vi "fasad.vi"(0 "Data In":T4, 2 "Display State In":T2, 3 "Container State":T3) -> (6 "Data Out":T4, 7 "Display State Out":T2, 8 "Action":T1)   [LabVIEW 2019, in "Visual.xctl"]
uses:
  Visual.xctl
  data.ctl
  <vilib>/_xctls/Container State.ctl
  state.ctl
  <vilib>/_xctls/Action.ctl
  <vilib>/express/express analysis/Spectral/Block/exnSpectralBlock spectral measurements RMS poly.vi
  <vilib>/express/express analysis/Spectral/Block/exnSpectralBlock spectral measurements RMS WFM.vi
  <vilib>/express/express analysis/Spectral/XNode/ExpressSpectralMeasurementsBlockNode.xnode
  <vilib>/_xctls/XControlSupport.lvlib
panel:
  in  "Tab Control":enum32{"Page 1", "Page 2"}(tab)
  out "Digital Waveform Graph":digitalwaveform(graph)
  out "Analyzer":cluster{"f0":dbl, "df":dbl, "magnitude":dbl[]}(graph)
  out "Osciloscope":waveform(dbl)(graph)
  in  "Tree":string(tree)
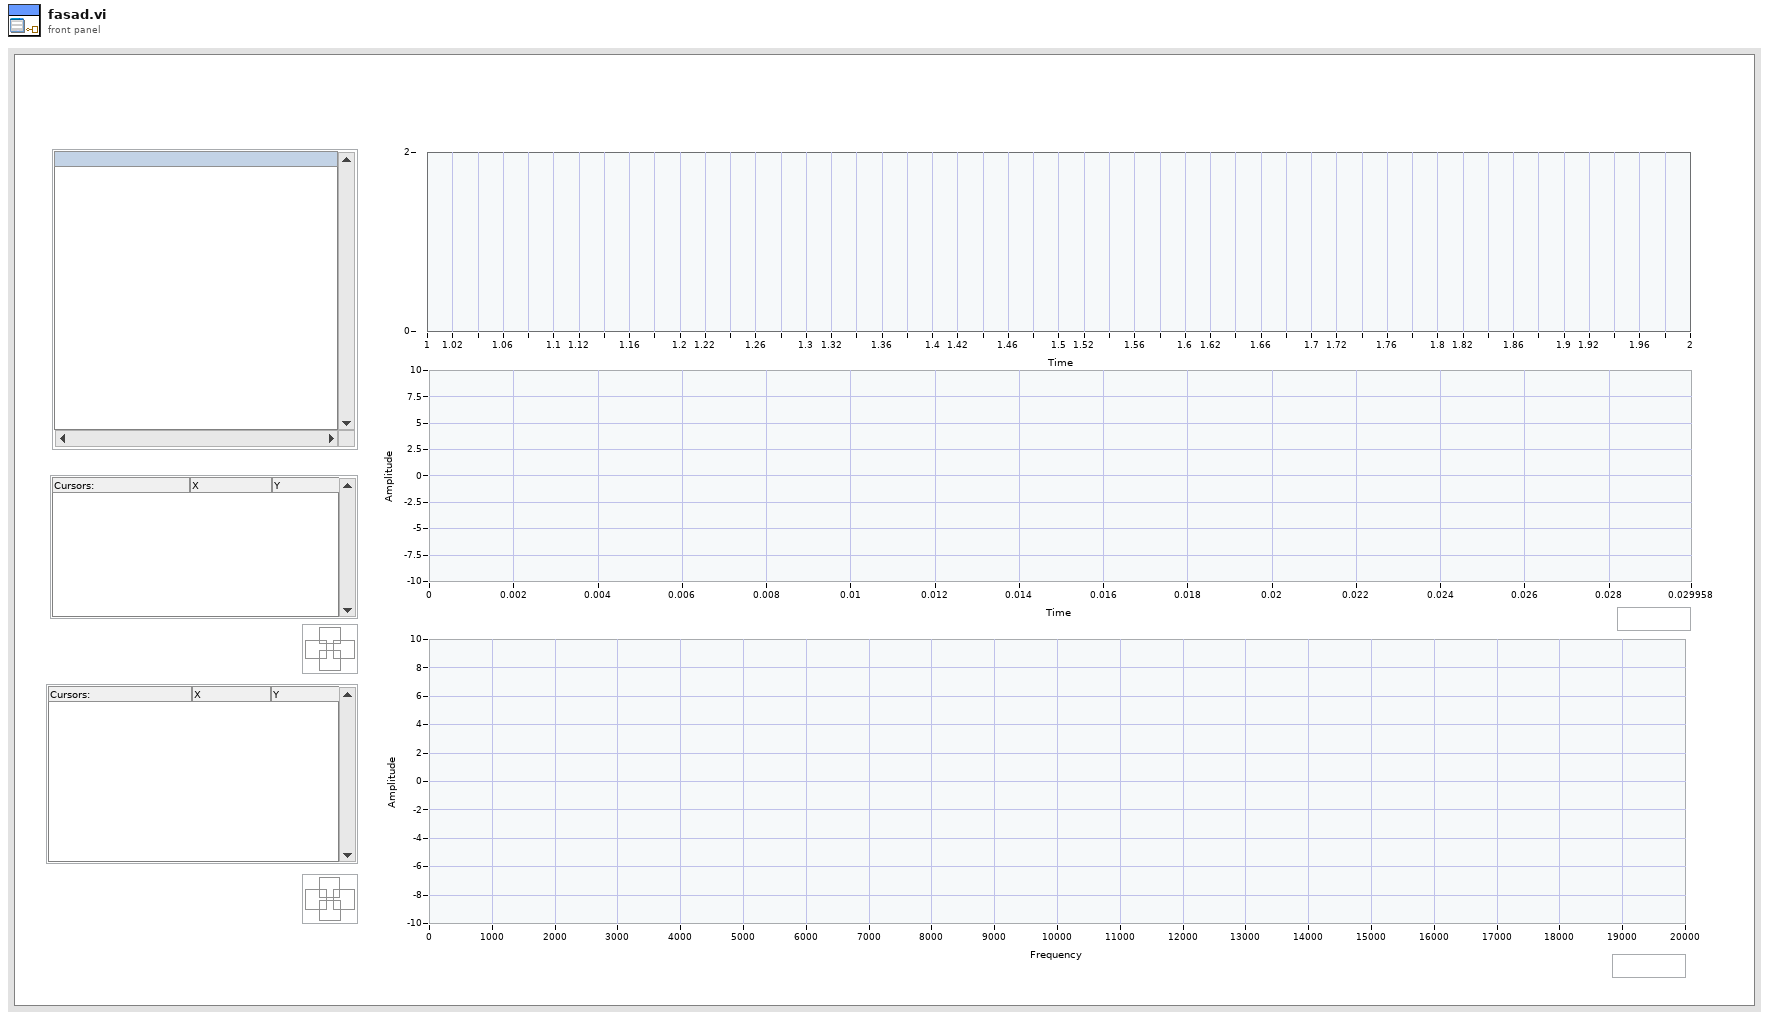
[diagram p1: front panel]
types:
  T1 = typedef "XControlSupport.lvlib/Action.ctl" = cluster{"Data Changed?":bool, "State Changed?":bool, "Action Name":string}
  T2 = typedef "Visual.xctl/state.ctl" = cluster{"Tree":string}
  T3 = typedef "XControlSupport.lvlib/Container State.ctl" = cluster{"Indicator?":bool, "Run Mode?":bool, " Refnum":refnum<vi>}
  T4 = typedef "Visual.xctl/data.ctl" = cluster{"Notes":string[], "Frame":u8[]}
  T5 = cluster{"averaging mode":u16, "weighting mode":u16, "number of averages":u32}
  T6 = cluster{"dB On (F)":bool, "unwrap phase (F)":bool, "convert to degree (F)":bool}
  T7 = enum8{"Enabled", "Disabled", "Disabled and Grayed Out"}
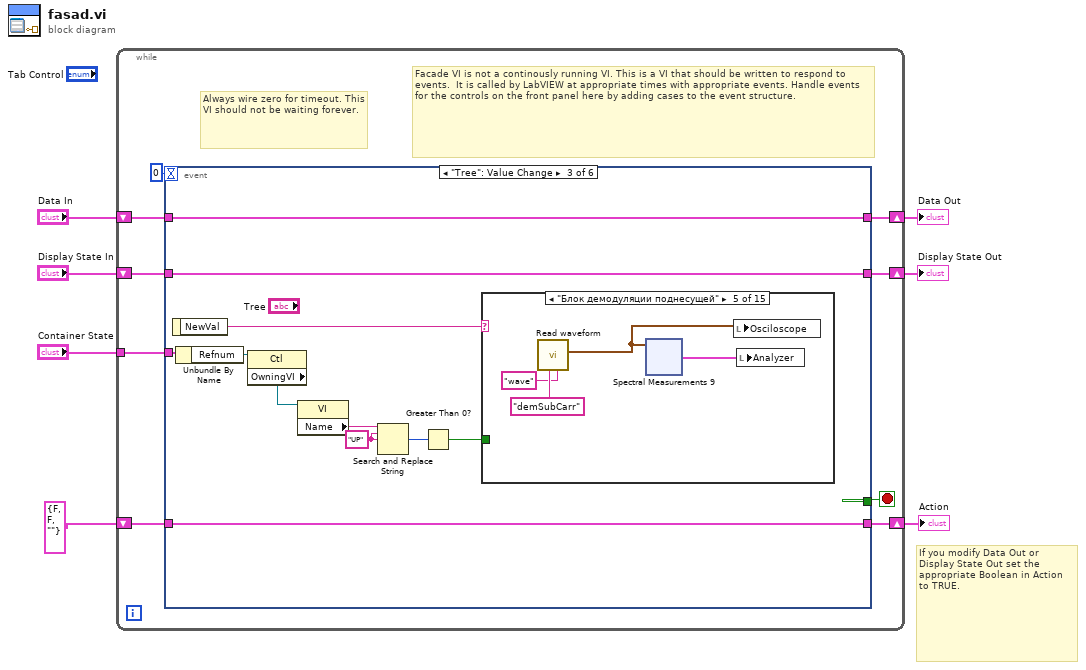
[diagram p0: block diagram]
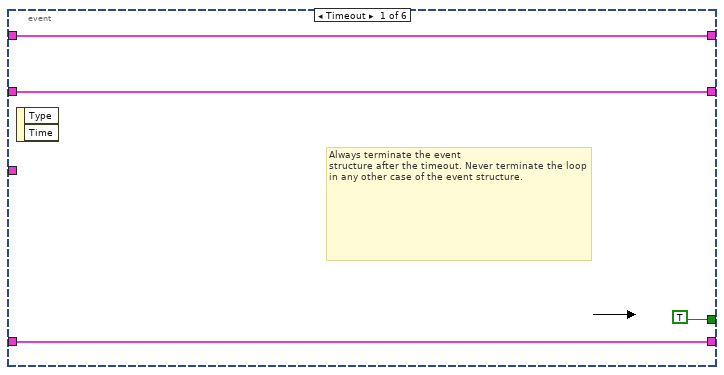
[diagram p2: hidden frame]
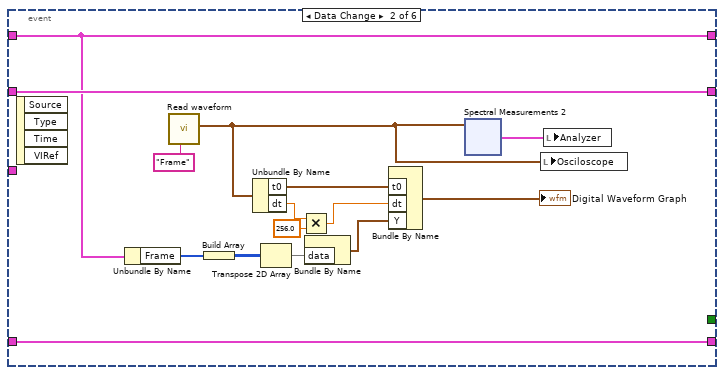
[diagram p3: hidden frame]
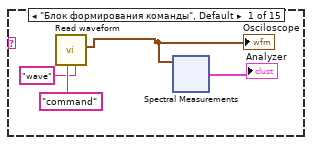
[diagram p4: hidden frame]
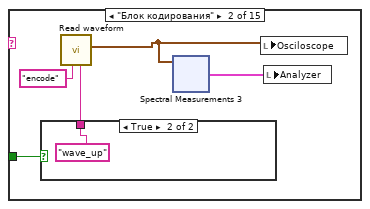
[diagram p5: hidden frame]
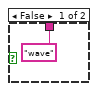
[diagram p6: hidden frame]
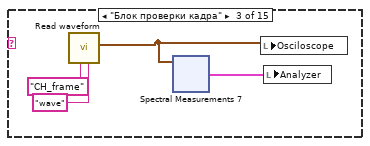
[diagram p7: hidden frame]
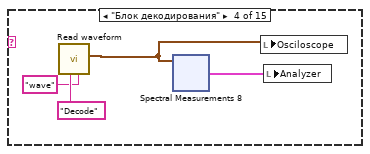
[diagram p8: hidden frame]
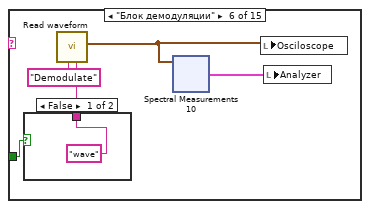
[diagram p9: hidden frame]
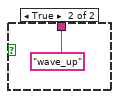
[diagram p10: hidden frame]
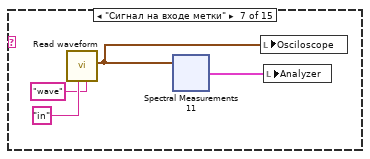
[diagram p11: hidden frame]
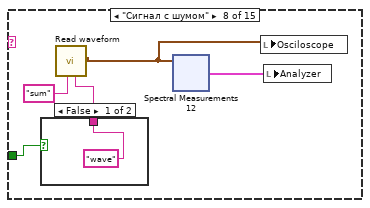
[diagram p12: hidden frame]
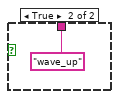
[diagram p13: hidden frame]
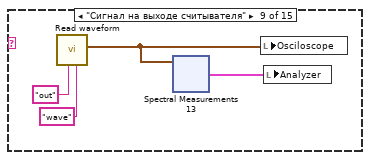
[diagram p14: hidden frame]
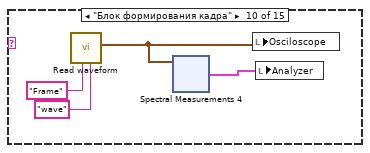
[diagram p15: hidden frame]
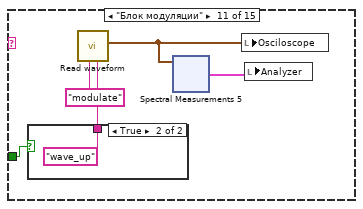
[diagram p16: hidden frame]
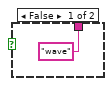
[diagram p17: hidden frame]
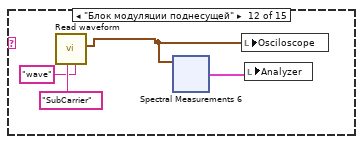
[diagram p18: hidden frame]
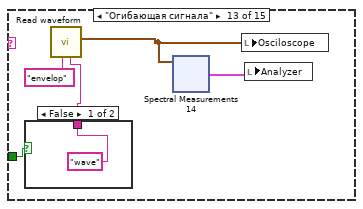
[diagram p19: hidden frame]
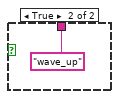
[diagram p20: hidden frame]
diagram:
  # "If you modify Data Out or\nDisplay State Out set the\nappropriate Boolean in Action\nto TRUE."
  n1 = while {
    shift-right: [w15] -> w4
    shift-left: "Display State In" -> [w16]
    tunnel: "Container State" -> [w12]
    shift-right: [w10] -> w7
    shift-left: "Data In" -> [w11]
    shift-right: [w8] -> w2
    shift-left: T1 {"Data Changed?"=FALSE, "State Changed?"=FALSE, "Action Name"=""} ("Action") -> [w9]
    stop <- w14 stop-if-true
    # "Facade VI is not a continously running VI. This is a VI that should be written to respond to events.  It is called by LabVIEW at appropriate times with appropriate events. Handle events for the controls on the front panel here by adding cases to the event structure."
    # "Always wire zero for timeout. This\nVI should not be waiting forever."
    n2 = event shown="[2] \"Tree\": Value Change" {
      selector: _ -> [_ _ _ _ _ _]
      dyn-events: _ -> [_ _ _ _ _ _]
      timeout: 0 -> [_ _ _ _ _ _]
      tunnel: w16 -> [w18 w35 w54 w282 w288 w306]
      tunnel: [w18 w35 w54 w282 w288 w306] -> w15
      tunnel: [TRUE _ _ _ _ _] -> w14
      tunnel: w12 -> [_ _ w52 _ w289 w297]
      tunnel: w11 -> [w17 w31 w55 w284 w286 w299]
      tunnel: [w17 w31 w55 w284 w286 w299] -> w10
      tunnel: [w19 w34 w56 w283 w287 w305] -> w8
      tunnel: w9 -> [w19 w34 w56 w283 w287 w305]
      event Timeout {
        # "Always terminate the event\nstructure after the timeout. Never terminate the loop in any other case of the event structure."
        n3 = event-data() -> ()  [unwired: 1 in, 2 out]
      }
      event Data Change {
        n4 = event-data() -> ()  [unwired: 1 in, 4 out]
        n5 = Unbundle By Name(w31) -> ("Frame"=w28:u8[])
        n6 = call "Read waveform.vi"("Note"="Frame") -> ("waveform out"=w27:waveform(dbl))  [unwired: 9 in, 1 out]
        n7 = Build Array(w28) -> (w30:u8[][])
        n8 = Unbundle By Name(w27) -> ("t0"=w26:timestamp, "dt"=w23:dbl)
        n9 = Transpose 2D Array(2D array=w30) -> (transposed array=w29:u8[][])
        n10 = Multiply(x=w23, y=256.0) -> (x*y=w22:dbl)
        n11 = Bundle By Name("data"=w29) -> (w25:digitaldata)  [unwired: 1 in]
        n12 = Bundle By Name("t0"=w26, "dt"=w22, "Y"=w25) -> (→"Digital Waveform Graph":digitalwaveform)  [unwired: 1 in]
        n13 = xnode ("Spectral Measurements 2")("Signals"=w27) -> ("FFT - (RMS)"=w33:cluster{"f0":dbl, "df":dbl, "magnitude":dbl[]})  [unwired: 1 in, 2 out]
        n14 = local write "Osciloscope"(w27) -> ()
        n15 = local write "Analyzer"(w33) -> ()
      }
      event "Tree": Value Change {
        w48 = "UP" ("replace string (\"\")")
        n16 = event-data() -> ("NewVal"=w53:string)  [unwired: 1 in]
        n17 = Unbundle By Name(w52) -> ("Refnum"=w51:refnum<vi>)
        n18 = property class="Ctl"(reference=w51) -> ("OwningVI"=w47:refnum<vi>)  [unwired: 1 in, 2 out]
        n19 = property class="VI"(reference=w47) -> ("Name"=w50:string)  [unwired: 1 in, 2 out]
        n20 = Search and Replace String(input string=w50, search string=w48, replace string=w48) -> (number of replacements=w49:i32)  [unwired: 5 in, 3 out]
        n21 = Greater Than 0?(x=w49) -> (x > 0?=w46:bool)
        n22 = case shown="\"Блок демодуляции поднесущей\"" w53 {
          tunnel: w46 -> [_ w71 _ _ _ w130 _ w161 _ _ w206 _ w238 _ _]
          frame "Блок формирования команды", Default {
            n23 = call "Read waveform.vi"("Channel"="wave", "Note"="command") -> ("waveform out"=w57:waveform(dbl))  [unwired: 8 in, 1 out]
            "Osciloscope" <- w57
            n24 = xnode ("Spectral Measurements")("Signals"=w57) -> ("FFT - (RMS)"=→"Analyzer":cluster{"f0":dbl, "df":dbl, "magnitude":dbl[]})  [unwired: 1 in, 2 out]
          }
          frame "Блок кодирования" {
            n25 = case shown="True" w71 {
              tunnel: ["wave" ("Channel") "wave_up" ("Channel")] -> w72
              frame False {
              }
              frame True {
              }
            }
            n26 = call "Read waveform.vi"("Channel"=w72, "Note"="encode") -> ("waveform out"=w73:waveform(dbl))  [unwired: 8 in, 1 out]
            n27 = xnode ("Spectral Measurements 3")("Signals"=w73) -> ("FFT - (RMS)"=w75:cluster{"f0":dbl, "df":dbl, "magnitude":dbl[]})  [unwired: 1 in, 2 out]
            n28 = local write "Osciloscope"(w73) -> ()
            n29 = local write "Analyzer"(w75) -> ()
          }
          frame "Блок проверки кадра" {
            n30 = call "Read waveform.vi"("Channel"="wave", "Note"="CH_frame") -> ("waveform out"=w89:waveform(dbl))  [unwired: 8 in, 1 out]
            n31 = xnode ("Spectral Measurements 7")("Signals"=w89) -> ("FFT - (RMS)"=w91:cluster{"f0":dbl, "df":dbl, "magnitude":dbl[]})  [unwired: 1 in, 2 out]
            n32 = local write "Osciloscope"(w89) -> ()
            n33 = local write "Analyzer"(w91) -> ()
          }
          frame "Блок декодирования" {
            n34 = call "Read waveform.vi"("Channel"="wave", "Note"="Decode") -> ("waveform out"=w103:waveform(dbl))  [unwired: 8 in, 1 out]
            n35 = xnode ("Spectral Measurements 8")("Signals"=w103) -> ("FFT - (RMS)"=w105:cluster{"f0":dbl, "df":dbl, "magnitude":dbl[]})  [unwired: 1 in, 2 out]
            n36 = local write "Osciloscope"(w103) -> ()
            n37 = local write "Analyzer"(w105) -> ()
          }
          frame "Блок демодуляции поднесущей" {
            n38 = call "Read waveform.vi"("Channel"="wave", "Note"="demSubCarr") -> ("waveform out"=w117:waveform(dbl))  [unwired: 8 in, 1 out]
            n39 = xnode ("Spectral Measurements 9")("Signals"=w117) -> ("FFT - (RMS)"=w119:cluster{"f0":dbl, "df":dbl, "magnitude":dbl[]})  [unwired: 1 in, 2 out]
            n40 = local write "Osciloscope"(w117) -> ()
            n41 = local write "Analyzer"(w119) -> ()
          }
          frame "Блок демодуляции" {
            n42 = case shown="False" w130 {
              tunnel: ["wave" ("Channel") "wave_up" ("Channel")] -> w131
              frame False {
              }
              frame True {
              }
            }
            n43 = call "Read waveform.vi"("Channel"=w131, "Note"="Demodulate") -> ("waveform out"=w132:waveform(dbl))  [unwired: 8 in, 1 out]
            n44 = xnode ("Spectral Measurements 10")("Signals"=w132) -> ("FFT - (RMS)"=w134:cluster{"f0":dbl, "df":dbl, "magnitude":dbl[]})  [unwired: 1 in, 2 out]
            n45 = local write "Osciloscope"(w132) -> ()
            n46 = local write "Analyzer"(w134) -> ()
          }
          frame "Сигнал на входе метки" {
            n47 = call "Read waveform.vi"("Channel"="wave", "Note"="in") -> ("waveform out"=w149:waveform(dbl))  [unwired: 8 in, 1 out]
            n48 = xnode ("Spectral Measurements 11")("Signals"=w149) -> ("FFT - (RMS)"=w150:cluster{"f0":dbl, "df":dbl, "magnitude":dbl[]})  [unwired: 1 in, 2 out]
            n49 = local write "Osciloscope"(w149) -> ()
            n50 = local write "Analyzer"(w150) -> ()
          }
          frame "Сигнал с шумом" {
            n51 = case shown="False" w161 {
              tunnel: ["wave" ("Channel") "wave_up" ("Channel")] -> w162
              frame False {
              }
              frame True {
              }
            }
            n52 = call "Read waveform.vi"("Channel"=w162, "Note"="sum") -> ("waveform out"=w164:waveform(dbl))  [unwired: 8 in, 1 out]
            n53 = xnode ("Spectral Measurements 12")("Signals"=w164) -> ("FFT - (RMS)"=w165:cluster{"f0":dbl, "df":dbl, "magnitude":dbl[]})  [unwired: 1 in, 2 out]
            n54 = local write "Osciloscope"(w164) -> ()
            n55 = local write "Analyzer"(w165) -> ()
          }
          frame "Сигнал на выходе считывателя" {
            n56 = call "Read waveform.vi"("Channel"="wave", "Note"="out") -> ("waveform out"=w180:waveform(dbl))  [unwired: 8 in, 1 out]
            n57 = xnode ("Spectral Measurements 13")("Signals"=w180) -> ("FFT - (RMS)"=w181:cluster{"f0":dbl, "df":dbl, "magnitude":dbl[]})  [unwired: 1 in, 2 out]
            n58 = local write "Osciloscope"(w180) -> ()
            n59 = local write "Analyzer"(w181) -> ()
          }
          frame "Блок формирования кадра" {
            n60 = call "Read waveform.vi"("Channel"="wave", "Note"="Frame") -> ("waveform out"=w194:waveform(dbl))  [unwired: 8 in, 1 out]
            n61 = xnode ("Spectral Measurements 4")("Signals"=w194) -> ("FFT - (RMS)"=w195:cluster{"f0":dbl, "df":dbl, "magnitude":dbl[]})  [unwired: 1 in, 2 out]
            n62 = local write "Osciloscope"(w194) -> ()
            n63 = local write "Analyzer"(w195) -> ()
          }
          frame "Блок модуляции" {
            n64 = case shown="True" w206 {
              tunnel: ["wave" ("Channel") "wave_up" ("Channel")] -> w207
              frame False {
              }
              frame True {
              }
            }
            n65 = call "Read waveform.vi"("Channel"=w207, "Note"="modulate") -> ("waveform out"=w209:waveform(dbl))  [unwired: 8 in, 1 out]
            n66 = xnode ("Spectral Measurements 5")("Signals"=w209) -> ("FFT - (RMS)"=w210:cluster{"f0":dbl, "df":dbl, "magnitude":dbl[]})  [unwired: 1 in, 2 out]
            n67 = local write "Osciloscope"(w209) -> ()
            n68 = local write "Analyzer"(w210) -> ()
          }
          frame "Блок модуляции поднесущей" {
            n69 = call "Read waveform.vi"("Channel"="wave", "Note"="SubCarrier") -> ("waveform out"=w224:waveform(dbl))  [unwired: 8 in, 1 out]
            n70 = xnode ("Spectral Measurements 6")("Signals"=w224) -> ("FFT - (RMS)"=w226:cluster{"f0":dbl, "df":dbl, "magnitude":dbl[]})  [unwired: 1 in, 2 out]
            n71 = local write "Osciloscope"(w224) -> ()
            n72 = local write "Analyzer"(w226) -> ()
          }
          frame "Огибающая сигнала" {
            n73 = case shown="False" w238 {
              tunnel: ["wave" ("Channel") "wave_up" ("Channel")] -> w237
              frame False {
              }
              frame True {
              }
            }
            n74 = call "Read waveform.vi"("Channel"=w237, "Note"="envelop") -> ("waveform out"=w239:waveform(dbl))  [unwired: 8 in, 1 out]
            n75 = xnode ("Spectral Measurements 14")("Signals"=w239) -> ("FFT - (RMS)"=w241:cluster{"f0":dbl, "df":dbl, "magnitude":dbl[]})  [unwired: 1 in, 2 out]
            n76 = local write "Osciloscope"(w239) -> ()
            n77 = local write "Analyzer"(w241) -> ()
          }
          frame "Сигнал на входе считывателя" {
            n78 = call "Read waveform.vi"("Channel"="wave_up", "Note"="in") -> ("waveform out"=w255:waveform(dbl))  [unwired: 8 in, 1 out]
            n79 = xnode ("Spectral Measurements 15")("Signals"=w255) -> ("FFT - (RMS)"=w257:cluster{"f0":dbl, "df":dbl, "magnitude":dbl[]})  [unwired: 1 in, 2 out]
            n80 = local write "Osciloscope"(w255) -> ()
            n81 = local write "Analyzer"(w257) -> ()
          }
          frame "Сигнал на выходе метки" {
            n82 = call "Read waveform.vi"("Channel"="wave_up", "Note"="out") -> ("waveform out"=w269:waveform(dbl))  [unwired: 8 in, 1 out]
            n83 = xnode ("Spectral Measurements 16")("Signals"=w269) -> ("FFT - (RMS)"=w271:cluster{"f0":dbl, "df":dbl, "magnitude":dbl[]})  [unwired: 1 in, 2 out]
            n84 = local write "Osciloscope"(w269) -> ()
            n85 = local write "Analyzer"(w271) -> ()
          }
        }
      }
      event Display State Change {
        n86 = event-data() -> ()  [unwired: 1 in, 4 out]
      }
      event Direction Change {
        n87 = event-data() -> ()  [unwired: 1 in, 4 out]
        n88 = Unbundle By Name(w289) -> ("Indicator?"=w285:bool)
        n89 = case shown="True" w285 {
          frame False {
            n90 = property on="Tree" class="Tree (strict)"("Allow Editing Cells"=TRUE) -> ()  [unwired: 2 in, 2 out]
          }
          frame True {
            n91 = property on="Tree" class="Tree (strict)"("Allow Editing Cells"=FALSE) -> ()  [unwired: 2 in, 2 out]
          }
        }
      }
      event Exec State Change {
        w292 = "UP" ("replace string (\"\")")
        n92 = event-data() -> ()  [unwired: 1 in, 4 out]
        n93 = Unbundle By Name(w297) -> ("Run Mode?"=w304:bool)
        n94 = Unbundle By Name(w297) -> ("Refnum"=w296:refnum<vi>)
        n95 = property class="Ctl"(reference=w296) -> ("OwningVI"=w298:refnum<vi>)  [unwired: 1 in, 2 out]
        n96 = property class="VI"(reference=w298) -> ("Name"=w295:string)  [unwired: 1 in, 2 out]
        n97 = Select(t=T7."Enabled" ("Disabled"), s=w304, f=T7."Disabled" ("Disabled")) -> (s? t:f=w301:T7)
        n98 = Search and Replace String(input string=w295, search string=w292, replace string=w292) -> (number of replacements=w294:i32)  [unwired: 5 in, 3 out]
        n99 = Greater Than 0?(x=w294) -> (x > 0?=w293:bool)
        n100 = control-ref of="Tree"() -> (w300:refnum<vi>)
        n101 = property on="Osciloscope" class="WFGraph (strict)"("DisabledEnum"=w301) -> ()  [unwired: 2 in, 2 out]
        n102 = property on="Tree" class="Tree (strict)"("DisabledEnum"=w301) -> ()  [unwired: 2 in, 2 out]
        n103 = property on="Analyzer" class="WFGraph (strict)"("DisabledEnum"=w301) -> ()  [unwired: 2 in, 2 out]
        n104 = call "Init_tree.vi"("First Call?: T/F"=w293, "TreeControl in"=w300) -> ()  [unwired: 10 in]
      }
    }
  }
  "Display State Out" <- w4
  "Data Out" <- w7
  "Action" <- w2
